vi "Untitled 1.vi"() -> ()   [LabVIEW 2020]
panel:
  out "String 2":string
  out "String":string
  in  "Keyboard":T1
  in  "ENTER":bool
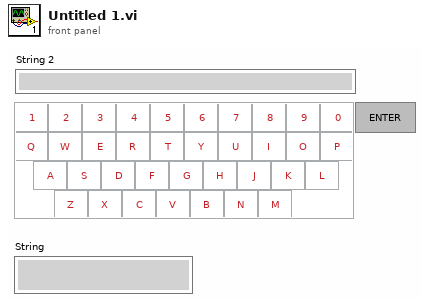
[diagram p1: front panel]
types:
  T1 = cluster{"Q":bool, "W":bool, " E":bool, "R":bool, "T":bool, "Y":bool, "U":bool, "I":bool, "O":bool, "P":bool, "A":bool, "S":bool, "D":bool, "F":bool, "G":bool, "H":bool, "J":bool, "K":bool, "L":bool, "Z":bool, "X":bool, "C":bool, "V":bool, "B":bool, "N":bool, "M":bool, "1":bool, "2":bool, "3":bool, "4":bool, "5":bool, "6":bool, "7":bool, "8":bool, "9":bool, "0":bool}
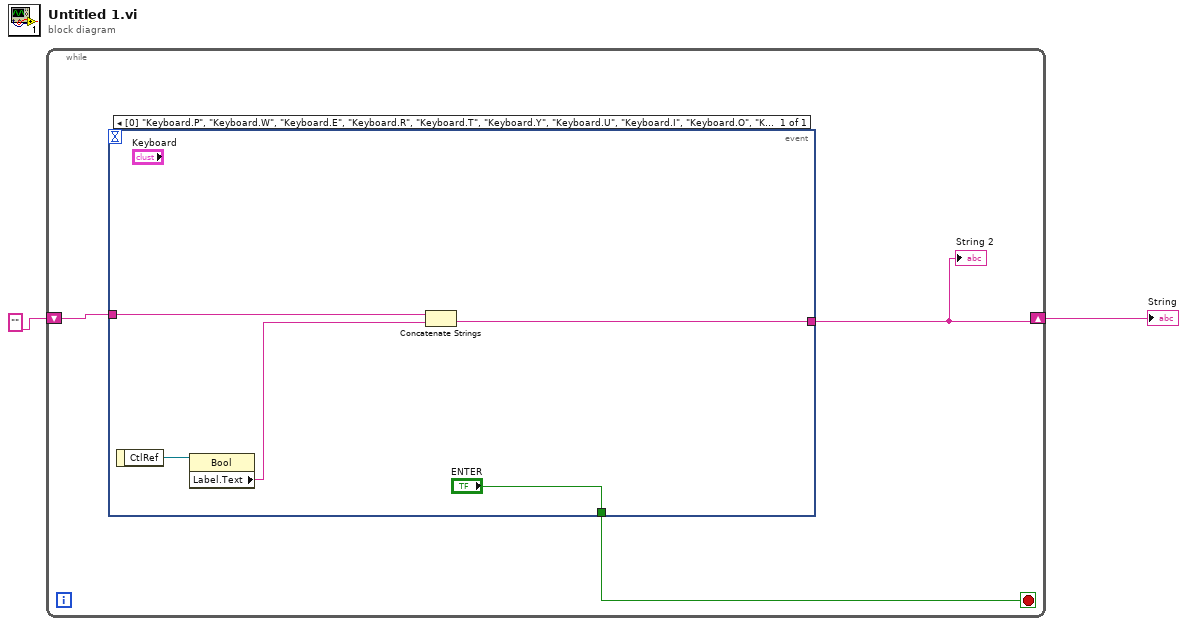
[diagram p0: block diagram]
diagram:
  n1 = while {
    shift-right: [w4] -> w1
    shift-left: "" -> [w5]
    stop <- w3 stop-if-true
    n2 = event shown="[0] \"Keyboard.P\", \"Keyboard.W\", \"Keyboard.E\", \"Keyboard.R\", \"Keyboard.T\", \"Keyboard.Y\", \"Keyboard.U\", \"Keyboard.I\", \"Keyboard.O\", \"Keyboard.A\", \"Keyboard.S\", \"Keyboard.D\", \"Keyboard.F\", \"Keyboard.G\", \"Keyboard.H\", \"Keyboard.J\", \"Keyboard.K\", \"Keyboard.L\", \"Keyboard.Z\", \"Keyboard.X\", \"Keyboard.C\", \"Keyboard.V\", \"Keyboard.B\", \"Keyboard.N\", \"Keyboard.M\", \"Keyboard.1\", \"Keyboard.2\", \"Keyboard.3\", \"Keyboard.4\", \"Keyboard.6\", \"Keyboard.7\", \"Keyboard.8\", \"Keyboard.9\", \"Keyboard.0\", \"ENTER\": Value Change" {
      selector: _ -> [_]
      dyn-events: _ -> [_]
      timeout: _ -> [_]
      tunnel: [w8] -> w4
      tunnel: w5 -> [w7]
      tunnel: ["ENTER"] -> w3
      event "Keyboard.P", "Keyboard.W", "Keyboard.E", "Keyboard.R", "Keyboard.T", "Keyboard.Y", "Keyboard.U", "Keyboard.I", "Keyboard.O", "Keyboard.A", "Keyboard.S", "Keyboard.D", "Keyboard.F", "Keyboard.G", "Keyboard.H", "Keyboard.J", "Keyboard.K", "Keyboard.L", "Keyboard.Z", "Keyboard.X", "Keyboard.C", "Keyboard.V", "Keyboard.B", "Keyboard.N", "Keyboard.M", "Keyboard.1", "Keyboard.2", "Keyboard.3", "Keyboard.4", "Keyboard.6", "Keyboard.7", "Keyboard.8", "Keyboard.9", "Keyboard.0", "ENTER": Value Change {
        n3 = event-data() -> ("CtlRef"=w10:refnum<vi>)  [unwired: 1 in]
        n4 = property class="Bool"(reference=w10) -> ("Label.Text"=w9:string)  [unwired: 1 in, 2 out]
        n5 = Concatenate Strings(w7, w9) -> (w8:string)
      }
    }
    "String 2" <- w4
  }
  "String" <- w1
